vi "getFilePattern.vi"(8 "error in (no error)":errorcluster, 11 "MS-Word in":refnum<class "MS-Word.lvclass">) -> (0 "error out":errorcluster, 1 "pattern":string, 2 "pattern label":string, 3 "MS-Word out":refnum<class "MS-Word.lvclass">)   [LabVIEW 2017, in "LabVIEW NPOI.lvlib" / "MS-Word.lvclass"]
doc: "Private method to get the <b>pattern lable</b> and the <b>pattern</b> from the <b>Docuement</b>.\n\nNote: \n<b>pattern lable</b>: is the label to display in the file dialog box next to the custom pattern.\n<b>pattern</b>: restricts the files displayed in the dialog box to those whose name matches pattern."
uses:
  MS-Word.lvclass
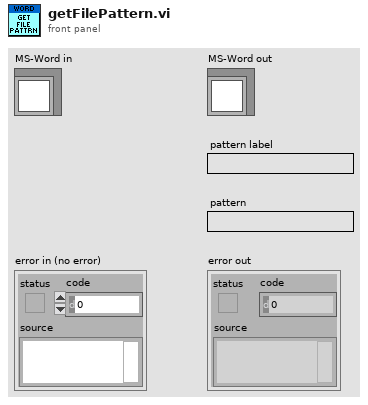
[diagram p1: front panel]
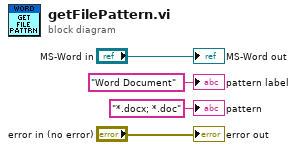
[diagram p0: block diagram]
diagram:
  "error out" <- "error in (no error)"
  "MS-Word out" <- "MS-Word in"
  "pattern" <- "*.docx; *.doc" ("pattern")
  "pattern label" <- "Word Document" ("pattern label")
